vi "Map Lookup Test.vi"() -> ()   [LabVIEW 2020, in "VectoScratch.lvlib"]
uses:
  VectoScratch.lvlib
panel:
  out "Waveform Chart":dbl(graph)
  out "Avg Array Time / lookup":dbl format="%#_6f"
  out "Array Lookup":i32[](array[numeric])
  out "Avg Map Time / lookup":dbl format="%#_6f"
  out "Map Lookup":i32[](array[numeric])
  in  "# Lookups":i32=1000
  in  "Word Length":i32=20
  in  "Words":i32=100
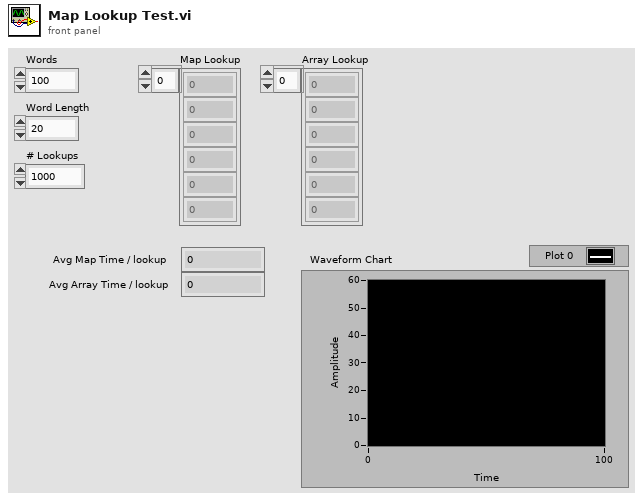
[diagram p1: front panel]
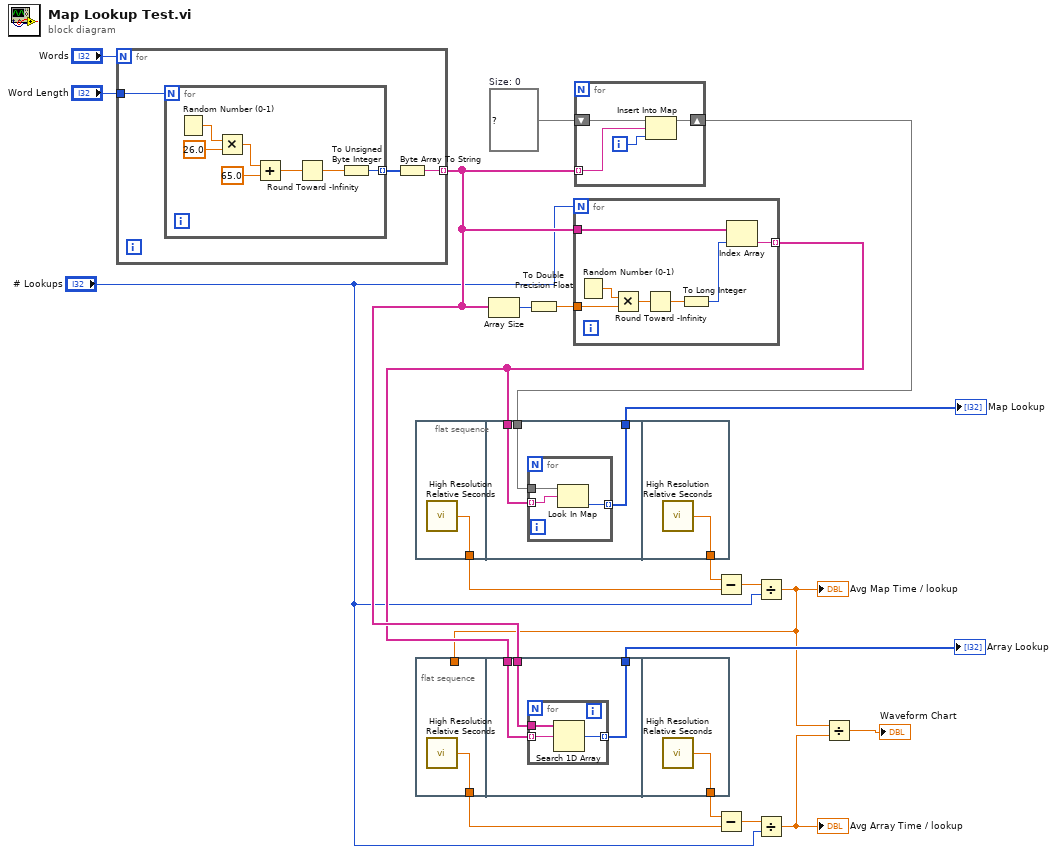
[diagram p0: block diagram]
diagram:
  w19 = map{string, i32} {}  # Size: 0
  n1 = for {
    N: "Words" -> [_]
    tunnel: [w22] -> w10 mode=indexing
    tunnel: "Word Length" -> [w21]
    n2 = for {
      N: w21 -> [_]
      tunnel: [w25] -> w23 mode=indexing
      n3 = Random Number (0-1)() -> (number: 0 to 1=w30:dbl)
      n4 = Multiply(x=w30, y=26.0) -> (x*y=w28:dbl)
      n5 = Add(x=w28, y=65.0) -> (x+y=w26:dbl)
      n6 = Round Toward -Infinity(1:w26) -> (0:w24:dbl)
      n7 = To Unsigned Byte Integer(number=w24) -> (unsigned 8bit integer=w25:u8)
    }
    n8 = Byte Array To String(unsigned byte array=w23) -> (string=w22:string)
  }
  n9 = flat-sequence {
    tunnel: [w31] -> w12
    tunnel: w15 -> [w34]
    tunnel: w9 -> [w33]
    tunnel: [w32] -> w14
    tunnel: [w38] -> w13
    frame #0 {
      n10 = call <vilib>:"High Resolution Relative Seconds.vi"() -> ("relative seconds"=w31:dbl)
    }
    frame #1 {
      n11 = for {
        tunnel: w34 -> [w37]
        tunnel: w33 -> [w36] mode=indexing
        tunnel: [w35] -> w32 mode=indexing
        n12 = Look In Map(map=w37, key=w36) -> (value=w35:i32)  [unwired: 1 in, 1 out]
      }
    }
    frame #2 {
      n13 = call <vilib>:"High Resolution Relative Seconds.vi"() -> ("relative seconds"=w38:dbl)
    }
  }
  n14 = flat-sequence {
    tunnel: [w39] -> w7
    tunnel: w3 -> [_]
    tunnel: w10 -> [w42]
    tunnel: w9 -> [w41]
    tunnel: [w40] -> w11
    tunnel: [w46] -> w8
    frame #0 {
      n15 = call <vilib>:"High Resolution Relative Seconds.vi"() -> ("relative seconds"=w39:dbl)
    }
    frame #1 {
      n16 = for {
        tunnel: w42 -> [w45]
        tunnel: w41 -> [w44] mode=indexing
        tunnel: [w43] -> w40 mode=indexing
        n17 = Search 1D Array(1D array=w45, element=w44) -> (index of element=w43:i32)  [unwired: 1 in]
      }
    }
    frame #2 {
      n18 = call <vilib>:"High Resolution Relative Seconds.vi"() -> ("relative seconds"=w46:dbl)
    }
  }
  n19 = Array Size(array=w10) -> (size(s)=w18:i32)
  n20 = To Double Precision Float(number=w18) -> (double precision float=w17:dbl)
  n21 = for {
    N: "# Lookups" -> [_]
    tunnel: w10 -> [w49]
    tunnel: w17 -> [w53]
    tunnel: [w47] -> w9 mode=indexing
    n22 = Random Number (0-1)() -> (number: 0 to 1=w52:dbl)
    n23 = Multiply(x=w52, y=w53) -> (x*y=w51:dbl)
    n24 = Round Toward -Infinity(1:w51) -> (0:w50:dbl)
    n25 = To Long Integer(number=w50) -> (32bit integer=w48:i32)
    n26 = Index Array(array=w49, index=w48) -> (element=w47:string)
  }
  n27 = for {
    tunnel: w10 -> [w56] mode=indexing
    shift-right: [w55] -> w15
    shift-left: w19 -> [w57]
    i -> [w54]
    n28 = Insert Into Map(map in=w57, key=w56, value=w54) -> (map out=w55:map{string, i32})  [unwired: 2 out]
  }
  n29 = Subtract(x=w13, y=w12) -> (x-y=w6:dbl)
  n30 = Subtract(x=w8, y=w7) -> (x-y=w5:dbl)
  n31 = Divide(x=w6, y="# Lookups") -> (x/y=w3:dbl)
  "Avg Map Time / lookup" <- w3
  n32 = Divide(x=w5, y="# Lookups") -> (x/y=w2:dbl)
  "Avg Array Time / lookup" <- w2
  n33 = Divide(x=w3, y=w2) -> (x/y=→"Waveform Chart":dbl)
  "Map Lookup" <- w14
  "Array Lookup" <- w11
